vi "Set Target Field.vi"(8 "error in":T2, 9 "Target Field (kG)":dbl format="%.3f", 11 "Communications Config":T1={"connection ID"=refnum, "IP"="192.168.0.108", "Active Comm Interface"=0, "Serial Port"="", "Programmer Type"=0, "connection ID"=refnum, "output cluster"={"GPIB address"=0, "GPIB bus"=0}} {"Programmer Type" items=["Model 430", "Model 420"]; "Active Comm Interface" items=["TCP/IP (Model 430 Only)", "RS232", "IEEE488"]}) -> (0 "error out":T2)   [LabVIEW 2017]
uses:
  commsControl.ctl
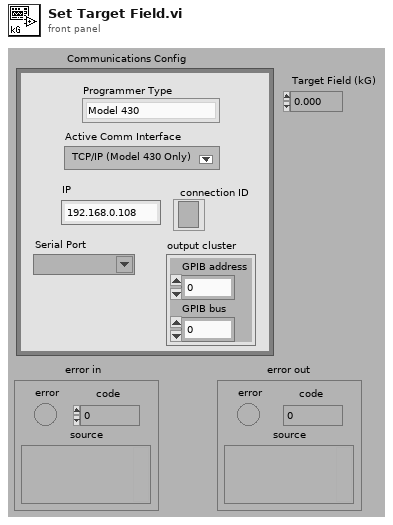
[diagram p1: front panel]
types:
  T1 = typedef "commsControl.ctl" = cluster{"connection ID":refnum<k5>, "IP":string, "Active Comm Interface":u16, "Serial Port":refnum<visa-resource-name>, "Programmer Type":u16, "connection ID":refnum<k5>, "output cluster":cluster{"GPIB address":i16, "GPIB bus":i16}}
  T2 = cluster{"error":bool, "code":i32, "source":string}
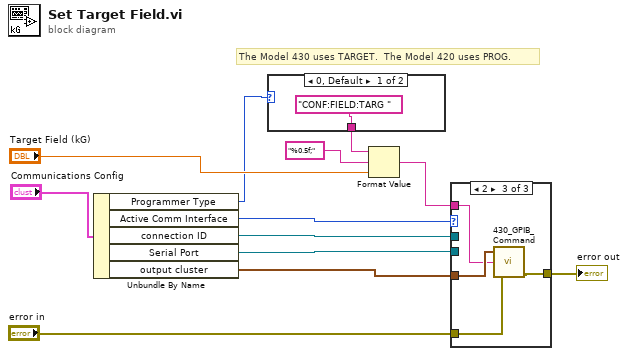
[diagram p0: block diagram]
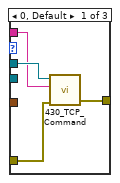
[diagram p2: hidden frame]
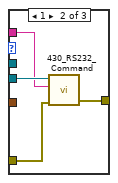
[diagram p3: hidden frame]
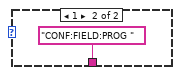
[diagram p4: hidden frame]
diagram:
  # "The Model 430 uses TARGET.  The Model 420 uses PROG."
  n1 = Unbundle By Name("Communications Config") -> ("Programmer Type"=w2:u16, "Active Comm Interface"=w4:u16, "connection ID"=w9:refnum<k5>, "Serial Port"=w8:refnum<visa-resource-name>, "output cluster"=w1:cluster{"GPIB address":i16, "GPIB bus":i16})
  n2 = case shown="0, Default" w2 {
    tunnel: ["CONF:FIELD:TARG " "CONF:FIELD:PROG "] -> w12
    frame 0, Default {
    }
    frame 1 {
    }
  }
  n3 = Format Value(string ("")=w12, format string="%0.5f;", value (0)="Target Field (kG)") -> (output string=w6:string)
  n4 = case shown="2" w4 {
    tunnel: [w18 w22 w26] -> w5
    tunnel: w1 -> [_ _ w25]
    tunnel: w9 -> [w17 _ _]
    tunnel: w8 -> [_ w21 _]
    tunnel: w6 -> [w16 w20 w24]
    tunnel: "error in" -> [w15 w19 w23]
    frame 0, Default {
      n5 = call "430_TCP_Command.vi"("error in (no error)"=w15, "Command"=w16, "connection ID"=w17) -> ("error out"=w18:errorcluster)  [unwired: 1 in, 2 out]
    }
    frame 1 {
      n6 = call "430_RS232_Command.vi"("error in (no error)"=w19, "Command"=w20, "VISA resource name"=w21) -> ("error out"=w22:errorcluster)  [unwired: 1 in, 2 out]
    }
    frame 2 {
      n7 = call "430_GPIB_Command.vi"("GPIB (In)"=w25, "Input command"=w24, "error in"=w23) -> ("error out"=w26:T2)  [unwired: 3 out]
    }
  }
  "error out" <- w5
